vi "SendDataEventData.vi"(7 "state in":T1, 8 "error in (no error)":errorcluster, 10 "message":T10, 11 "Qbus in":refnum<class "Qbus.lvclass">) -> (0 "error out":errorcluster)   [LabVIEW 2017, in "ServerComm.lvlib"]
uses:
  <vilib>/addons/InsightCM/Devices/Shared/Common/ServerComm/ServerComm.lvlib
  <vilib>/addons/InsightCM/MessageBus/Base/controls/Message.ctl
  <vilib>/addons/InsightCM/MessageBus/Base/controls/MessageHeader.ctl
  <vilib>/addons/InsightCM/MessageBus/Base/controls/KeyValuePair.ctl
  <vilib>/addons/InsightCM/Devices/Shared/Common/ServerComm/controls/config.ctl
  <vilib>/addons/InsightCM/MessageBus/TcpApi/controls/TcpMessageReference.ctl
  <vilib>/addons/InsightCM/MessageBus/Base/controls/ConnectionInfo.ctl
  <vilib>/addons/InsightCM/SRP/controls/DVR_data.ctl
  <vilib>/addons/InsightCM/SRP/controls/data.ctl
  <vilib>/addons/InsightCM/Devices/Shared/Common/ServerComm/controls/ConnectedStatusDvr.ctl
  <vilib>/addons/InsightCM/Devices/Shared/Common/ServerComm/controls/ConnectionStatus.ctl
  <vilib>/addons/InsightCM/Devices/Shared/Common/ServerComm/controls/DataSendStatus.ctl
  <vilib>/addons/InsightCM/Devices/Shared/Common/ServerComm/controls/DataSendMode.ctl
  <vilib>/addons/InsightCM/Devices/Shared/Common/ServerComm/controls/ReconnectData.ctl
  <vilib>/addons/InsightCM/Devices/Shared/Common/ServerComm/controls/ProvisioningVersionInfo.ctl
  <vilib>/addons/Qbus/Qbus.lvclass
  <vilib>/addons/InsightCM/MessageBus/MessageLibrary/DataStorage/controls/DataStorageSendDataEventRoutedMessageBody.ctl
  <vilib>/addons/InsightCM/MessageBus/Base/controls/DataEvent.ctl
  <vilib>/addons/InsightCM/MessageBus/Base/controls/DataSetMetadata.ctl
  <vilib>/addons/InsightCM/MessageBus/Base/controls/TrendPoint.ctl
  <vilib>/addons/InsightCM/MessageBus/Base/controls/TrendAlarmUpdate.ctl
  <vilib>/addons/InsightCM/MessageBus/Base/controls/TrendAlarmTransition.ctl
  <vilib>/addons/InsightCM/Devices/Shared/Common/ServerComm/controls/DataSendBody.ctl
  <vilib>/addons/InsightCM/MessageBus/Base/controls/IRoutingSource.ctl
  <vilib>/addons/InsightCM/Devices/Shared/Common/DataEvent/DataEvent.lvlib
  <vilib>/addons/InsightCM/SRP/SRP.lvlib
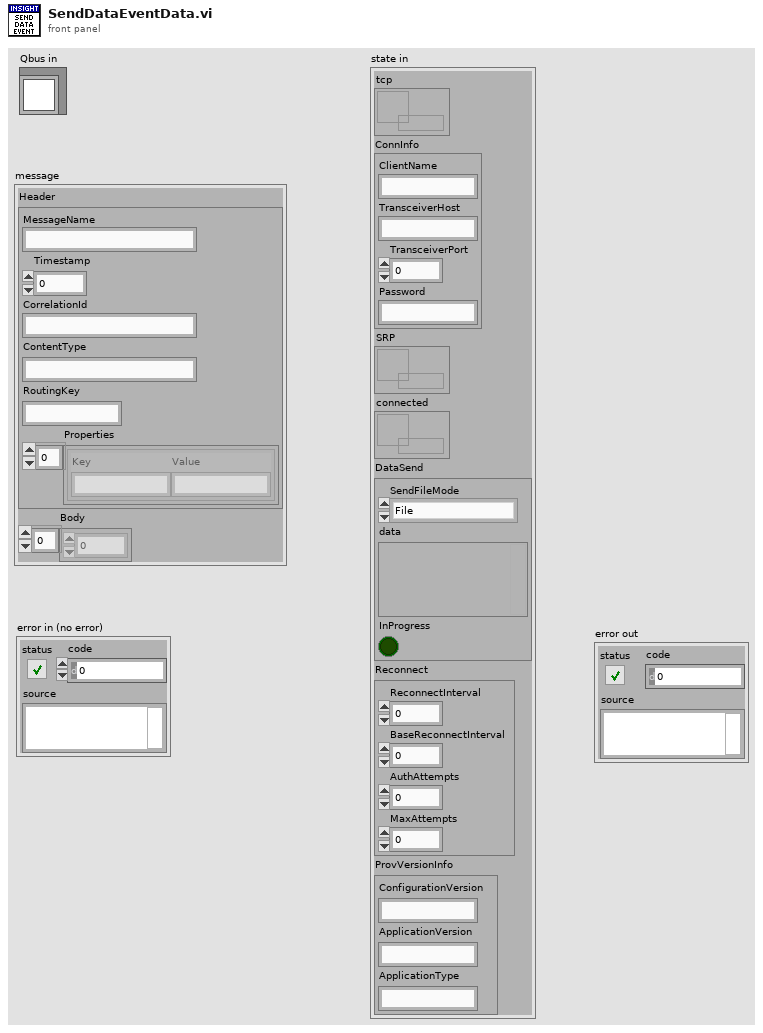
[diagram p1: front panel]
types:
  T1 = typedef "ServerComm.lvlib/config.ctl" = cluster{"tcp":T2, "ConnInfo":T3, "SRP":T4, "connected":T5, "DataSend":T6, "Reconnect":T8, "ProvVersionInfo":T9}
  T2 = typedef "TcpMessageReference.ctl" = refnum<data-value>
  T3 = typedef "ConnectionInfo.ctl" = cluster{"ClientName":string, "TransceiverHost":string, "TransceiverPort":u16, "Password":string}
  T4 = typedef "SRP.lvlib/DVR_data.ctl" = refnum<data-value>
  T5 = typedef "ServerComm.lvlib/ConnectedStatusDvr.ctl" = refnum<data-value>
  T6 = typedef "ServerComm.lvlib/DataSendStatus.ctl" = cluster{"SendFileMode":T7, "data":variant, "InProgress":bool}
  T7 = typedef "ServerComm.lvlib/DataSendMode.ctl" = enum16{"File", "InMemoryFile", "Stream", "StreamFileBlock", "ByteArray", "NoOp", "UnknownData"}
  T8 = typedef "ServerComm.lvlib/ReconnectData.ctl" = cluster{"ReconnectInterval":dbl, "BaseReconnectInterval":dbl, "AuthAttempts":i32, "MaxAttempts":i32}
  T9 = typedef "ServerComm.lvlib/ProvisioningVersionInfo.ctl" = cluster{"ConfigurationVersion":string, "ApplicationVersion":string, "ApplicationType":string}
  T10 = typedef "Message.ctl" = cluster{"Header":T11, "Body":u8[]}
  T11 = typedef "MessageHeader.ctl" = cluster{"MessageName":string, "Timestamp":i64, "CorrelationId":string, "ContentType":string, "RoutingKey":string, "Properties":T12[]}
  T12 = typedef "KeyValuePair.ctl" = cluster{"Key":string, "Value":string}
  T13 = typedef "ServerComm.lvlib/DataSendBody.ctl" = cluster{"tcp reference":T2, "SendFileMode":T7, "data":variant, "IRoutingSource":T14, "ReplyTo":string}
  T14 = typedef "IRoutingSource.ctl" = cluster{"CorrelationId":string, "ReplyTo":string}
  T15 = typedef "DataStorageSendDataEventRoutedMessageBody.ctl" = cluster{"DataEvent":T16, "DataSetMetadataList":T17[], "TrendPoints":T18[], "AlarmUpdates":T19[]}
  T16 = typedef "DataEvent.ctl" = cluster{"Id":string, "AssetNodeId":string, "Timestamp":i64, "Props":T12[]}
  T17 = typedef "DataSetMetadata.ctl" = cluster{"Id":string, "DataEventId":string, "AssetNodeId":string, "Type":string, "T0":i64, "Props":T12[]}
  T18 = typedef "TrendPoint.ctl" = cluster{"TrendPointId":string, "DataEventId":string, "Timestamp":i64, "Value":dbl, "Props":T12[]}
  T19 = typedef "TrendAlarmUpdate.ctl" = cluster{"RuleId":string, "Transition":T20}
  T20 = typedef "TrendAlarmTransition.ctl" = cluster{"At":i64, "Severity":i32, "Value":dbl, "Properties":T12[]}
  T21 = typedef "DataEvent.lvlib/EventReference.ctl" = refnum<data-value>
  T22 = typedef "DataEvent.lvlib/Event.ctl" = cluster{"DataEvent":T16, "DataSets":T23[], "TrendPoints":T18[], "Alarms":T19[]}
  T23 = typedef "DataEvent.lvlib/DataSet.ctl" = cluster{"DataSetMetadata":T17, "Values":sgl[], "Values DVR":refnum<data-value>}
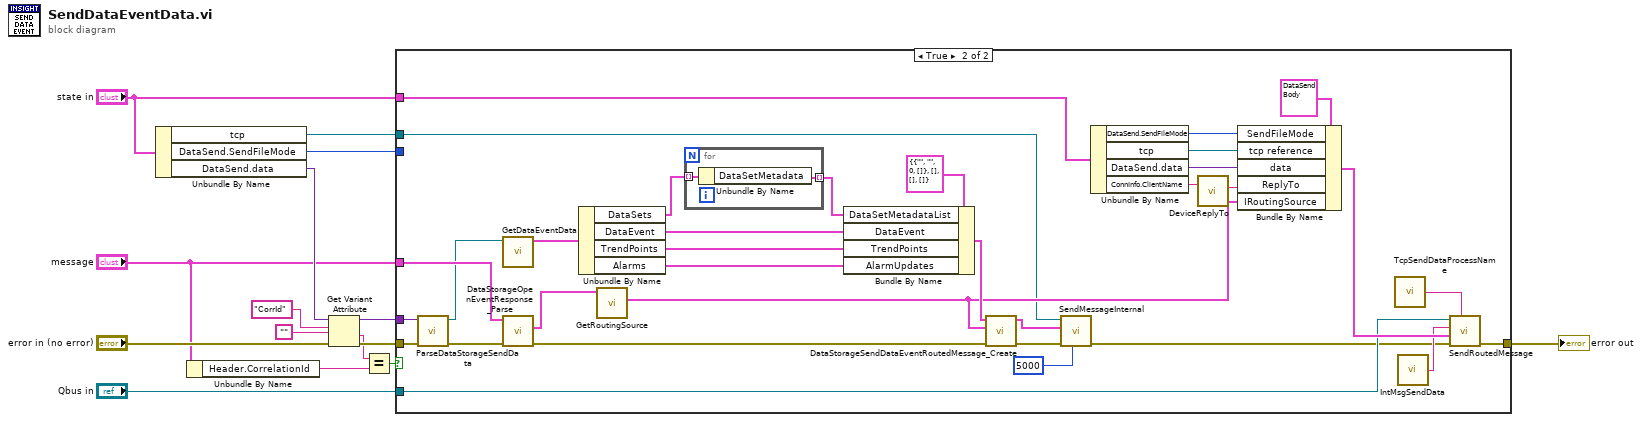
[diagram p0: block diagram]
diagram:
  n1 = Unbundle By Name("state in") -> ("tcp"=w15:T2, "DataSend.SendFileMode"=w4:T7, "DataSend.data"=w5:variant)
  n2 = Unbundle By Name("message") -> ("Header.CorrelationId"=w9:string)
  n3 = Get Variant Attribute(Variant=w5, name="CorrId", default value (empty Variant)="", error in="error in (no error)") -> (duplicate Variant=w13:variant, value=w8:string, error out=w12:errorcluster)  [unwired: 1 out]
  n4 = Equal?(x=w8, y=w9) -> (x = y?=w11:bool)
  n5 = case shown="True" w11 {
    tunnel: "Qbus in" -> [_ w23]
    tunnel: [w16 w27] -> w3
    tunnel: w4 -> [_ _]
    tunnel: "state in" -> [_ w25]
    tunnel: w12 -> [w16 w47]
    tunnel: w13 -> [_ w46]
    tunnel: "message" -> [_ w49]
    tunnel: w15 -> [_ w21]
    frame False {
    }
    frame True {
      n6 = call <vilib>:"ParseDataStorageSendData.vi"("error in (no error)"=w47, "body"=w46) -> ("error out"=w45:errorcluster, "event reference"=w43:T21)  [unwired: 4 in, 4 out]
      n7 = call <vilib>:"GetDataEventData.vi"("Data Value Reference in"=w43) -> ("Data"=w42:T22)  [unwired: 9 in, 1 out]
      n8 = call <vilib>:"DataStorageOpenEventResponse_Parse.vi"("error in (no error)"=w45, "Message"=w49) -> ("error out"=w44:errorcluster, "Header"=w48:T11)  [unwired: 7 in, 1 out]
      n9 = Unbundle By Name(w42) -> ("DataSets"=w38:T23[], "DataEvent"=w40:T16, "TrendPoints"=w39:T18[], "Alarms"=w22:T19[])
      n10 = call <vilib>:"GetRoutingSource.vi"("Header in"=w48) -> ("IRoutingSource"=w26:T14)  [unwired: 9 in, 1 out]
      n11 = for {
        tunnel: w38 -> [w51] mode=indexing
        tunnel: [w50] -> w37 mode=indexing
        n12 = Unbundle By Name(w51) -> ("DataSetMetadata"=w50:T17)
      }
      n13 = Bundle By Name(cluster=T15 {"DataEvent"={"Id"="", "AssetNodeId"="", "Timestamp"=0, "Props"=[]}, "DataSetMetadataList"=[], "TrendPoints"=[], "AlarmUpdates"=[]} ("Body"), "DataSetMetadataList"=w37, "DataEvent"=w40, "TrendPoints"=w39, "AlarmUpdates"=w22) -> (w36:T15)
      n14 = call <vilib>:"DataStorageSendDataEventRoutedMessage_Create.vi"("error in (no error)"=w44, "IRoutingSource"=w26, "DataStorageSendDataEventRoutedMessage"=w36) -> ("error out"=w18:errorcluster, "Message"=w20:T10)  [unwired: 7 in]
      n15 = call <vilib>:"SendMessageInternal.vi"("timeout (5 sec)"=5000, "error in (no error)"=w18, "message"=w20, "connection ID in"=w21) -> ("error out"=w17:errorcluster)  [unwired: 6 in, 1 out]
      n16 = Unbundle By Name(w25) -> ("DataSend.SendFileMode"=w24:T7, "tcp"=w31:T2, "DataSend.data"=w32:variant, "ConnInfo.ClientName"=w34:string)
      n17 = call <vilib>:"DeviceReplyTo.vi"("Device"=w34) -> ("ReplyTo"=w33:string)  [unwired: 10 in]
      n18 = Bundle By Name(cluster=T13 {"tcp reference"=refnum, "SendFileMode"=enum."File", "data"=variant, "IRoutingSource"={"CorrelationId"="", "ReplyTo"=""}, "ReplyTo"=""} ("DataSend"), "SendFileMode"=w24, "tcp reference"=w31, "data"=w32, "ReplyTo"=w33, "IRoutingSource"=w26) -> (w35:T13)
      n19 = call <vilib>:"TcpSendDataProcessName.vi"() -> ("process name"=w28:string)  [unwired: 5 in]
      n20 = call <vilib>:"IntMsgSendData.vi"() -> ("message name"=w29:string)  [unwired: 5 in]
      n21 = call <vilib>:"SendRoutedMessage.vi"("listener process"=w28, "error in (no error)"=w17, "message value"=w35, "message name"=w29, "Qbus in"=w23) -> ("error in (no error)"=w27:errorcluster)  [unwired: 5 in, 1 out]
    }
  }
  "error out" <- w3
